vi "(SubVI)_2Dstart_BD_ver16_transfering_MultiVesselsMultiDir_OnePatch.vi"(0 "Master Ctr (Ctr0)":tag, 1 "Master Ctr Terminal (PFI0)":tag, 2 "Galvo Hardware":T2, 3 "Camera Hardware":T1, 4 "input cluster":T3, 5 "error in (no error)":errorcluster, 6 "B-Scan Frequency":dbl=100.0, 7 "A-scans per Image":u32, 8 "Camera Delay (us)":dbl format="%.6f", 9 "A-scans per Cross Section":u32, 11 "Galvo Trigg per Cross Section":u32) -> (13 "Image Size":u32, 14 "Master Ctr Task Out":refnum<k21>, 15 "Galvo AO Task Out":refnum<k21>, 16 "Camera Ctr Task Out":refnum<k21>, 17 "Galvo Ctr Task Out":refnum<k21>, 18 "output cluster for DLL":T3, 19 "AO Err Out":errorcluster)   [LabVIEW 2019]
uses:
  <vilib>/DAQmx/write.llb/DAQmx Write (Analog 2D DBL NChan NSamp).vi
  <vilib>/DAQmx/create/channels.llb/DAQmx Create Channel (CO-Pulse Generation-Frequency).vi
  <vilib>/DAQmx/configure/timing.llb/DAQmx Timing (Implicit).vi
  <vilib>/DAQmx/configure/trigger.llb/DAQmx Start Trigger (Digital Edge).vi
  <vilib>/DAQmx/create/channels.llb/DAQmx Create Channel (AO-Voltage-Basic).vi
  <vilib>/DAQmx/configure/timing.llb/DAQmx Timing (Sample Clock).vi
  <vilib>/DAQmx/miscellaneous.llb/DAQmx Fill In Error Info.vi
  <resource>/objmgr/daqmx.rc
panel:
  out "B-Scan Frequency 2":dbl
  in  "counter":tag
  out "error out":errorcluster
  out "task out":refnum<k21>
  in  "2D frequency":i16
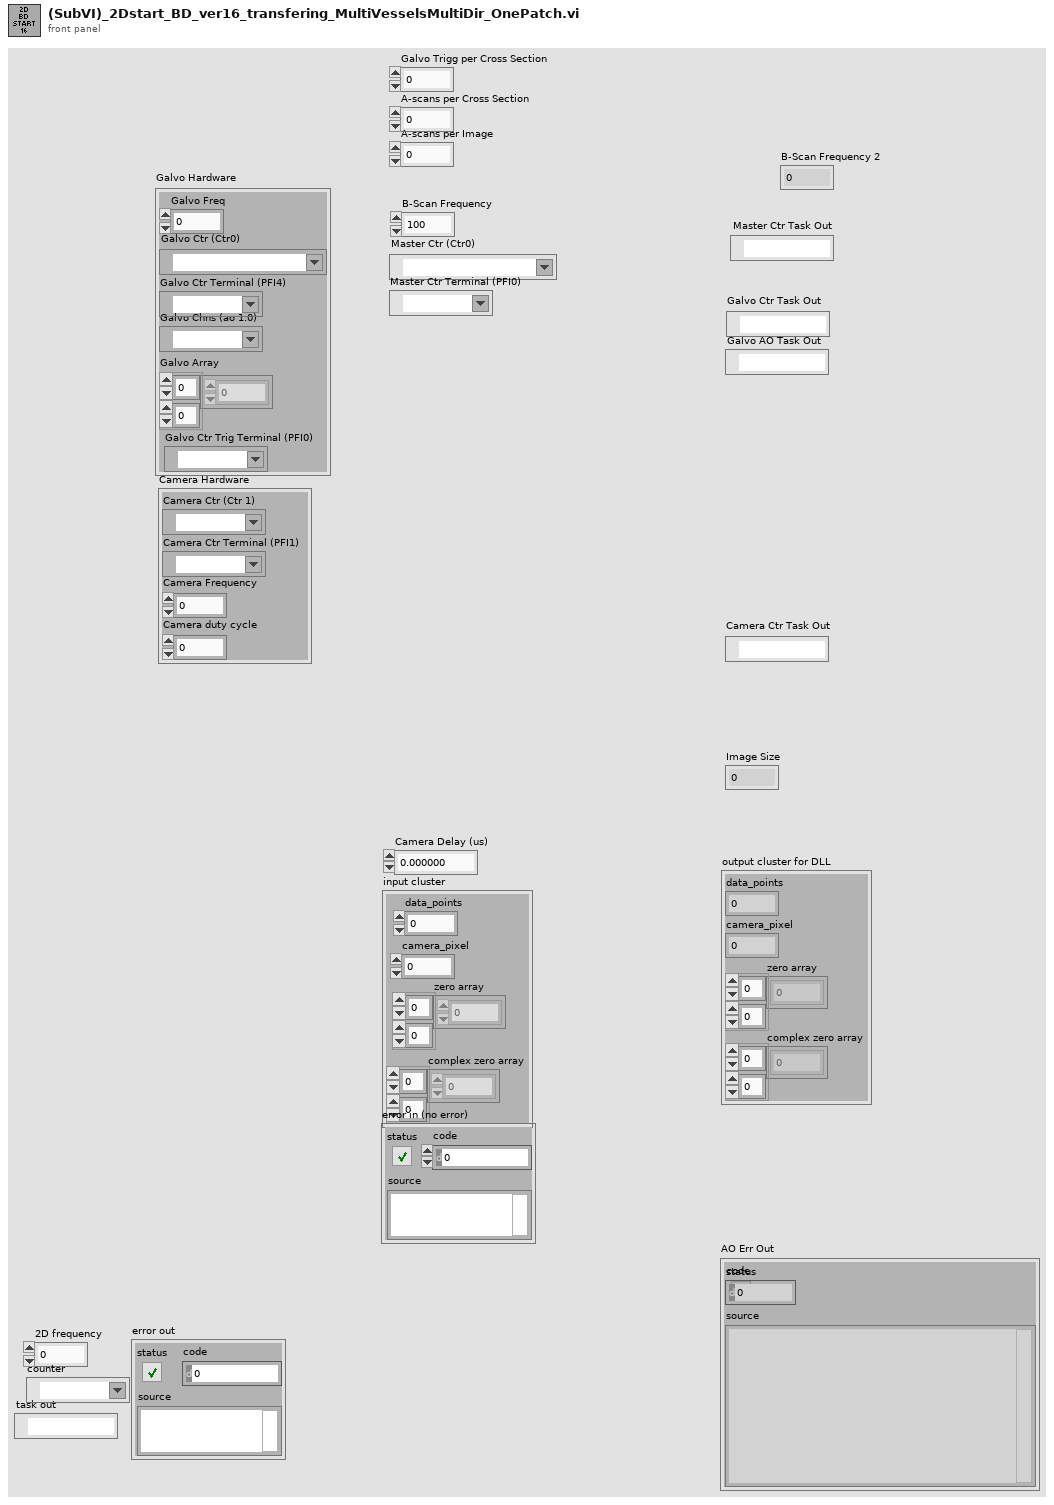
[diagram p1: front panel]
types:
  T1 = cluster{"Camera Ctr (Ctr 1)":tag, "Camera Ctr Terminal (PFI1)":tag, "Camera Frequency":dbl, "Camera duty cycle":dbl}
  T2 = cluster{"Galvo Array":dbl[][], "Galvo Chns (ao 1:0)":tag, "Galvo Ctr (Ctr0)":tag, "Galvo Ctr Terminal (PFI4)":tag, "Galvo Freq":dbl, "Galvo Ctr Trig Terminal (PFI0)":tag}
  T3 = cluster{"data_points":i32, "camera_pixel":i32, "zero array":dbl[][], "complex zero array":dbl[][]}
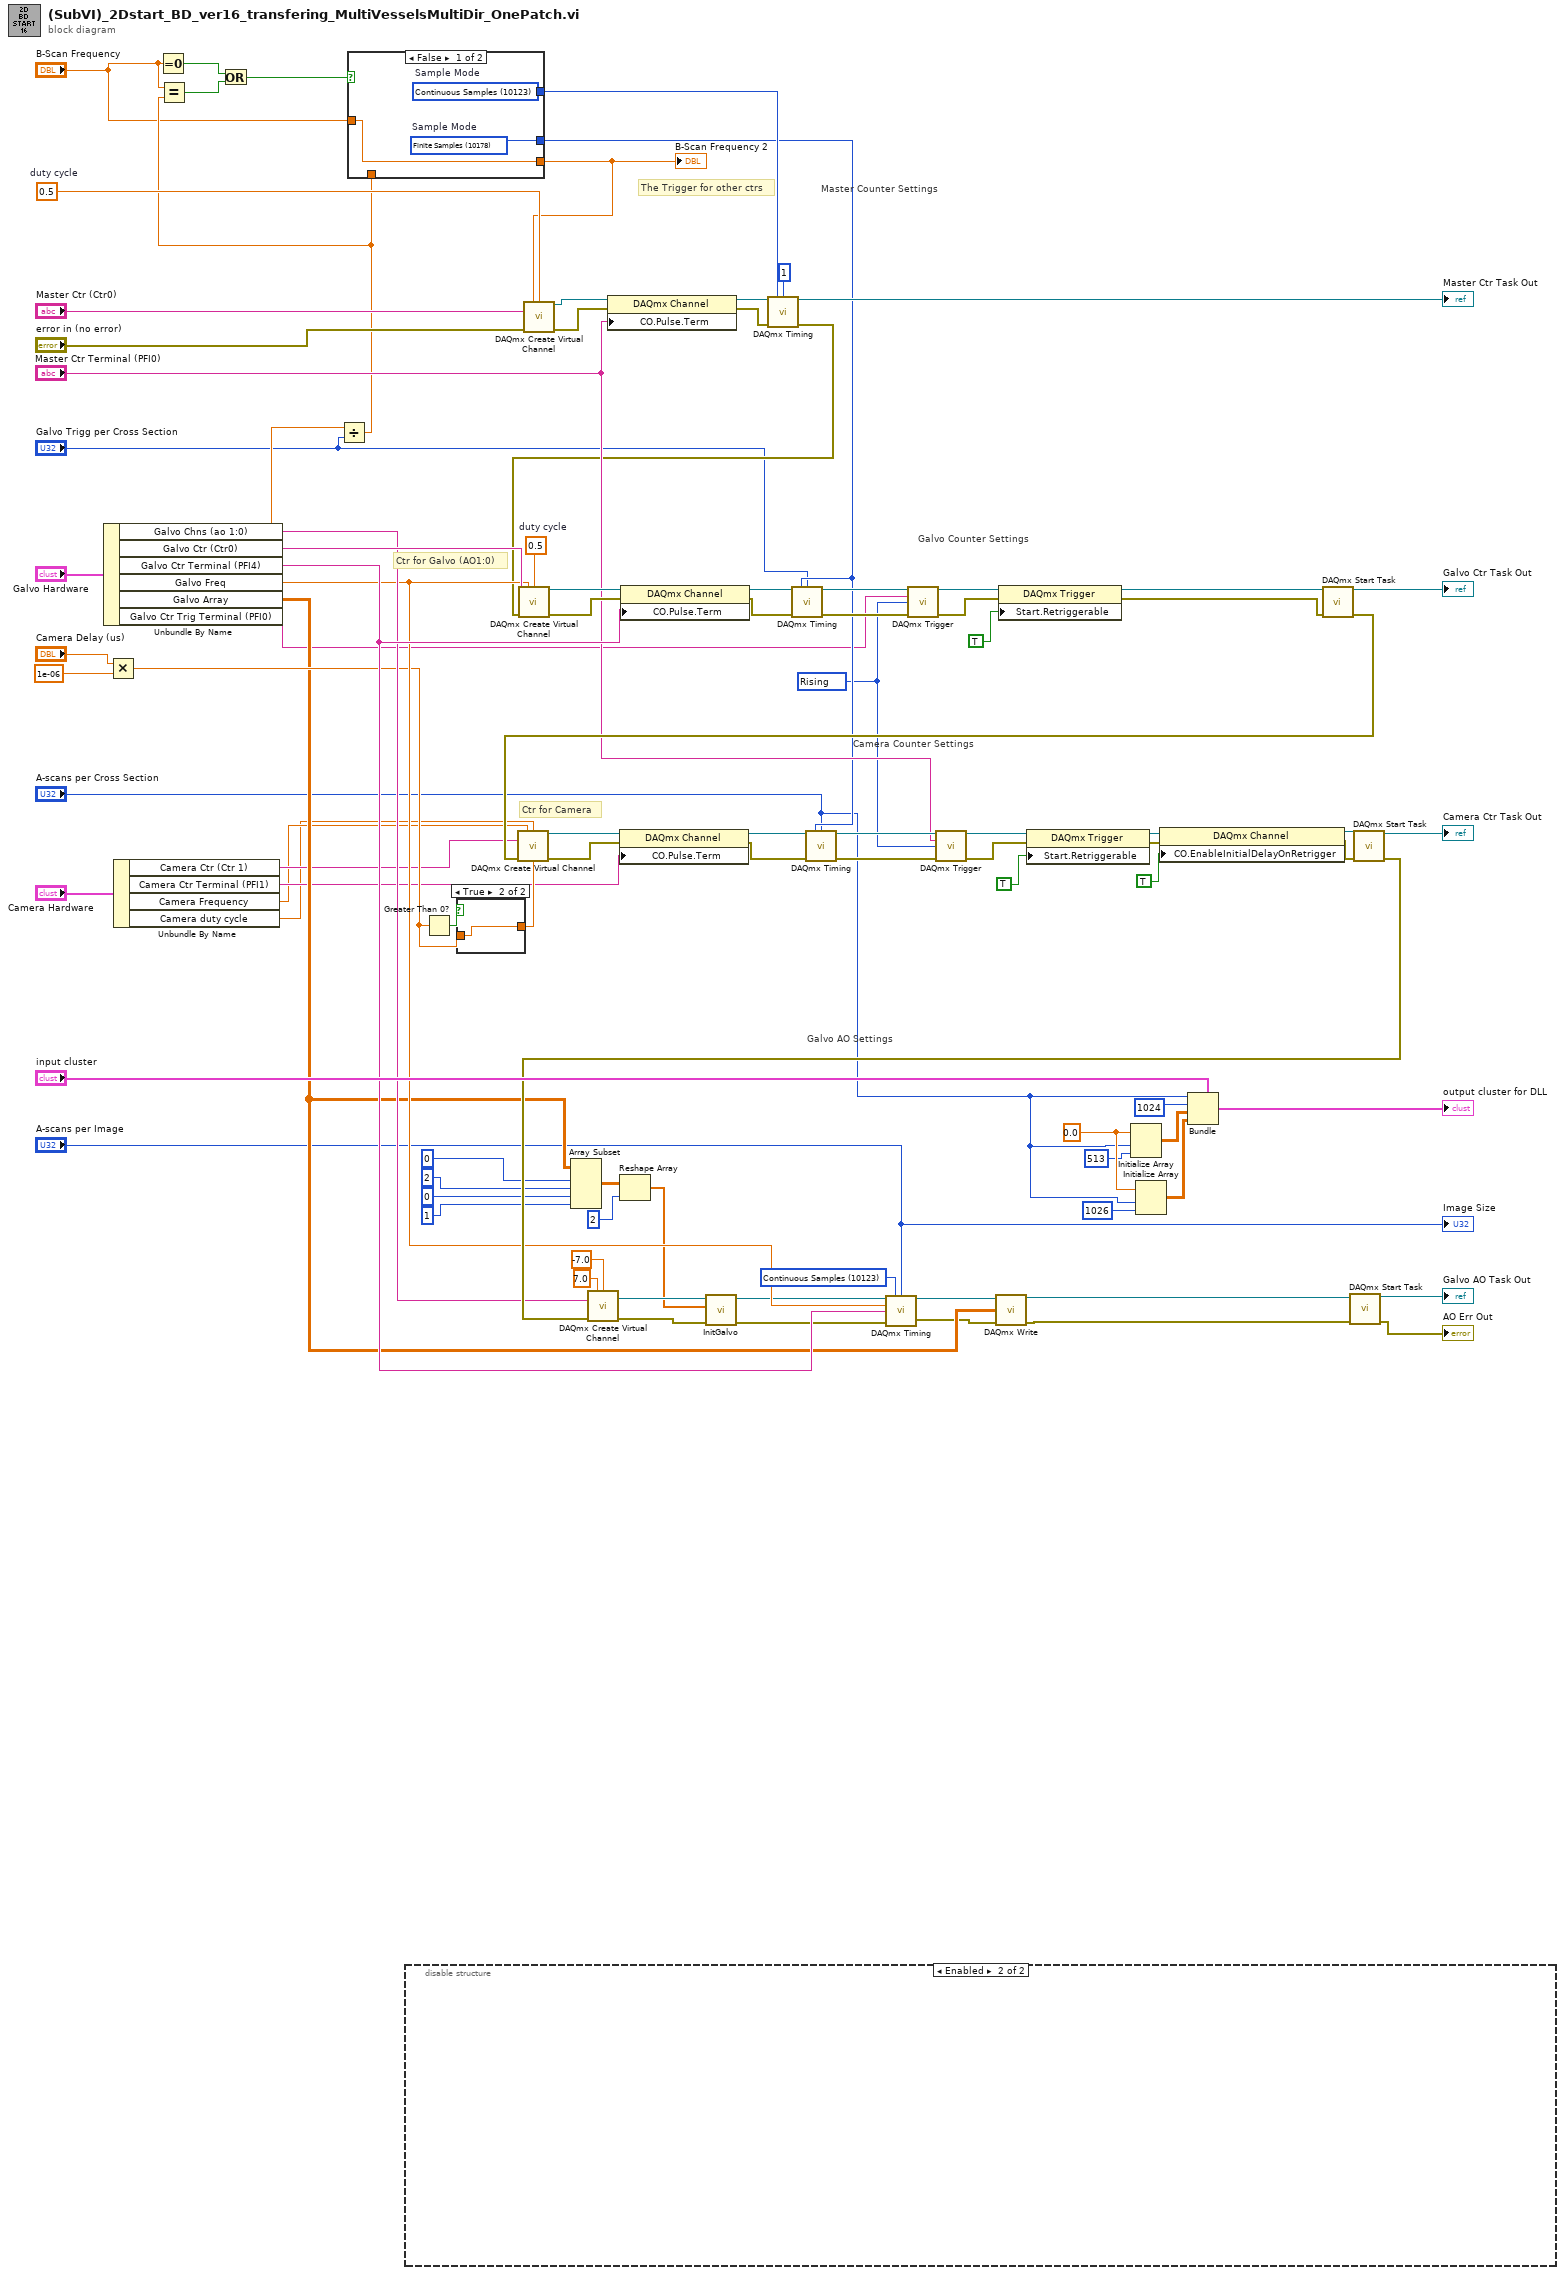
[diagram p0: block diagram]
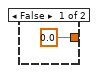
[diagram p2: hidden frame]
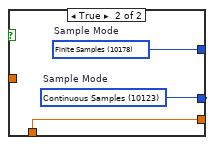
[diagram p3: hidden frame]
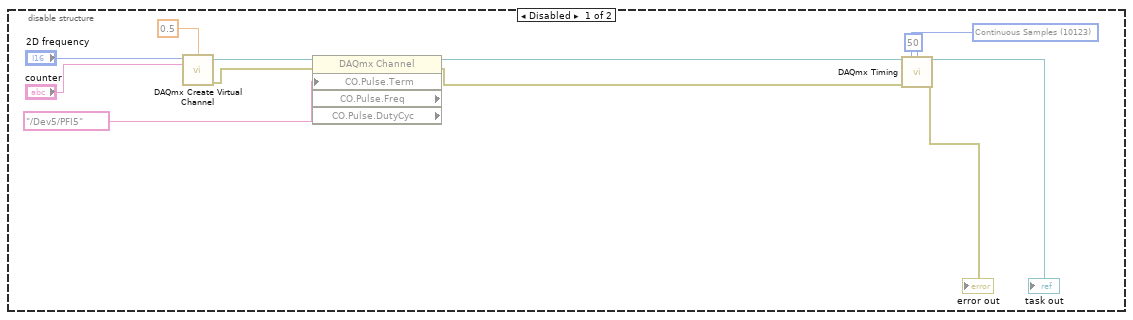
[diagram p4: hidden frame]
diagram:
  w27 = 0.0 ("element")
  w22 = 10123 items=["Finite Samples"=10178, "Continuous Samples"=10123, "Hardware Timed Single Point"=12522] ("sample mode")
  w46 = 10280 items=["Rising"=10280, "Falling"=10171] ("edge")
  w89 = 0.5  # duty cycle
  w94 = 0.5  # duty cycle
  # "Galvo AO Settings"
  # "Camera Counter Settings"
  # "Galvo Counter Settings"
  # "Master Counter Settings"
  # "Ctr for Camera"
  # "Ctr for Galvo (AO1:0)"
  # "The Trigger for other ctrs"
  n1 = Unbundle By Name("Galvo Hardware") -> ("Galvo Chns (ao 1:0)"=w66:tag, "Galvo Ctr (Ctr0)"=w68:tag, "Galvo Ctr Terminal (PFI4)"=w69:tag, "Galvo Freq"=w58:dbl, "Galvo Array"=w45:dbl[][], "Galvo Ctr Trig Terminal (PFI0)"=w7:tag)
  n2 = Multiply(x="Camera Delay (us)", y=1e-06) -> (x*y=w53:dbl)
  n3 = Unbundle By Name("Camera Hardware") -> ("Camera Ctr (Ctr 1)"=w43:tag, "Camera Ctr Terminal (PFI1)"=w42:tag, "Camera Frequency"=w41:dbl, "Camera duty cycle"=w40:dbl)
  n4 = Equal To 0?(x="B-Scan Frequency") -> (x = 0?=w37:bool)
  n5 = Divide(x=w58, y="Galvo Trigg per Cross Section") -> (x/y=w39:dbl)
  n6 = Equal?(x="B-Scan Frequency", y=w39) -> (x = y?=w36:bool)
  n7 = Or(x=w37, y=w36) -> (x .or. y?=w35:bool)
  n8 = case shown="False" w35 {
    tunnel: "B-Scan Frequency" -> [w101 _]
    tunnel: [w101 w104] -> w50
    tunnel: w39 -> [_ w104]
    tunnel: [w100 w103] -> w49
    tunnel: [w99 w102] -> w47
    frame False {
      w99 = 10178 items=["Finite Samples"=10178, "Continuous Samples"=10123, "Hardware Timed Single Point"=12522]  # Sample Mode
      w100 = 10123 items=["Finite Samples"=10178, "Continuous Samples"=10123, "Hardware Timed Single Point"=12522]  # Sample Mode
    }
    frame True {
      w102 = 10123 items=["Finite Samples"=10178, "Continuous Samples"=10123, "Hardware Timed Single Point"=12522]  # Sample Mode
      w103 = 10178 items=["Finite Samples"=10178, "Continuous Samples"=10123, "Hardware Timed Single Point"=12522]  # Sample Mode
    }
  }
  "B-Scan Frequency 2" <- w50
  n9 = disable-structure shown="Enabled" {
    frame Disabled {
      w113 = 10123 items=["Finite Samples"=10178, "Continuous Samples"=10123, "Hardware Timed Single Point"=12522] ("sample mode")
      n10 = call-poly <vilib>:"DAQmx Create Virtual Channel.vi"("frequency"="2D frequency", "duty cycle"=0.5, "counter"="counter") -> ("task out"=w109:refnum<k21>, "error out"=w108:errorcluster)  [unwired: 6 in, 5 out]
      n11 = property class="DAQmx Channel" props=["CO.Pulse.Term", "CO.Pulse.Freq", "CO.Pulse.DutyCyc"](reference=w109, error in=w108, "CO.Pulse.Term"=tag "/Dev5/PFI5") -> (reference out=w107:refnum<k21>, error out=w106:errorcluster)  [unwired: 2 out]
      n12 = call-poly <vilib>:"DAQmx Timing.vi"("task/channels in"=w107, "sample mode"=w113, "samples per channel"=50, "error in"=w106) -> ("task out"=→"task out":refnum<k21>, "error out"=→"error out":errorcluster)  [unwired: 2 in, 8 out]
    }
    frame Enabled {
    }
  }
  n13 = Greater Than 0?(x=w53) -> (x > 0?=w57:bool)
  n14 = case shown="True" w57 {
    tunnel: w53 -> [_ w118]
    tunnel: [0.0 ("Camera Delay") w118] -> w56
    frame False {
    }
    frame True {
    }
  }
  n15 = call-poly <vilib>:"DAQmx Create Virtual Channel.vi"("frequency"=w50, "duty cycle"=w94, "counter"="Master Ctr (Ctr0)", "error in"="error in (no error)") -> ("task out"=w97:refnum<k21>, "error out"=w96:errorcluster)  [unwired: 10 in]
  n16 = Array Subset(array=w45, index (row)=0 ("index"), length (row)=2 ("length"), index (col)=0 ("index"), length (col)=1 ("length")) -> (w17:dbl[][])
  n17 = property class="DAQmx Channel"(reference=w97, error in=w96, "CO.Pulse.Term"="Master Ctr Terminal (PFI0)") -> (reference out=w93:refnum<k21>, error out=w92:errorcluster)
  n18 = Reshape Array(w17, 2 ("dimension size")) -> (w12:dbl[])
  n19 = call-poly <vilib>:"DAQmx Timing.vi"("task/channels in"=w93, "sample mode"=w49, "samples per channel"=1, "error in"=w92) -> ("task out"=→"Master Ctr Task Out":refnum<k21>, "error out"=w52:errorcluster)  [unwired: 10 in]
  n20 = call-poly <vilib>:"DAQmx Create Virtual Channel.vi"("frequency"=w58, "duty cycle"=w89, "counter"=w68, "error in"=w52) -> ("task out"=w91:refnum<k21>, "error out"=w90:errorcluster)  [unwired: 10 in]
  n21 = property class="DAQmx Channel"(reference=w91, error in=w90, "CO.Pulse.Term"=w69) -> (reference out=w78:refnum<k21>, error out=w77:errorcluster)
  n22 = call-poly <vilib>:"DAQmx Timing.vi"("task/channels in"=w78, "sample mode"=w47, "samples per channel"="Galvo Trigg per Cross Section", "error in"=w77) -> ("task out"=w76:refnum<k21>, "error out"=w75:errorcluster)  [unwired: 10 in]
  n23 = call-poly <vilib>:"DAQmx Trigger.vi"("task/channels in"=w76, "source"=w7, "edge"=w46, "error in"=w75) -> ("task out"=w87:refnum<k21>, "error out"=w88:errorcluster)  [unwired: 10 in]
  n24 = property class="DAQmx Trigger"(reference=w87, error in=w88, "Start.Retriggerable"=TRUE) -> (reference out=w6:refnum<k21>, error out=w5:errorcluster)
  n25 = Initialize Array(w27, "A-scans per Cross Section", 513 ("dimension size")) -> (w25:dbl[][])
  n26 = Initialize Array(w27, "A-scans per Cross Section", 1026 ("dimension size")) -> (w26:dbl[][])
  n27 = Bundle(cluster="input cluster", "data_points"="A-scans per Cross Section", "camera_pixel"=1024, "zero array"=w25, "complex zero array"=w26) -> (→"output cluster for DLL":T3)
  n28 = call <vilib>:"DAQmx Start Task.vi"("task/channels in"=w6, "error in"=w5) -> ("task out"=→"Galvo Ctr Task Out":refnum<k21>, "error out"=w70:errorcluster)  [unwired: 12 in]
  n29 = call-poly <vilib>:"DAQmx Create Virtual Channel.vi"("frequency"=w41, "duty cycle"=w40, "counter"=w43, "error in"=w70, "initial delay"=w56) -> ("task out"=w84:refnum<k21>, "error out"=w83:errorcluster)  [unwired: 9 in]
  n30 = property class="DAQmx Channel"(reference=w84, error in=w83, "CO.Pulse.Term"=w42) -> (reference out=w74:refnum<k21>, error out=w73:errorcluster)
  n31 = call-poly <vilib>:"DAQmx Timing.vi"("task/channels in"=w74, "sample mode"=w47, "samples per channel"="A-scans per Cross Section", "error in"=w73) -> ("task out"=w72:refnum<k21>, "error out"=w71:errorcluster)  [unwired: 10 in]
  n32 = call-poly <vilib>:"DAQmx Trigger.vi"("task/channels in"=w72, "source"="Master Ctr Terminal (PFI0)", "edge"=w46, "error in"=w71) -> ("task out"=w81:refnum<k21>, "error out"=w82:errorcluster)  [unwired: 10 in]
  n33 = property class="DAQmx Trigger"(reference=w81, error in=w82, "Start.Retriggerable"=TRUE) -> (reference out=w64:refnum<k21>, error out=w63:errorcluster)
  n34 = property class="DAQmx Channel"(reference=w64, error in=w63, "CO.EnableInitialDelayOnRetrigger"=TRUE) -> (reference out=w61:refnum<k21>, error out=w60:errorcluster)
  n35 = call <vilib>:"DAQmx Start Task.vi"("task/channels in"=w61, "error in"=w60) -> ("task out"=→"Camera Ctr Task Out":refnum<k21>, "error out"=w67:errorcluster)  [unwired: 12 in]
  n36 = call-poly <vilib>:"DAQmx Create Virtual Channel.vi"("maximum value"=7.0, "minimum value"=-7.0, "physical channels"=w66, "error in"=w67) -> ("task out"=w13:refnum<k21>, "error out"=w16:errorcluster)  [unwired: 5 in, 5 out]
  n37 = call "InitGalvo.vi"("error in"=w16, "Output Array"=w12, "task/channels in"=w13) -> ("error out"=w15:errorcluster, "task out"=w14:refnum<k21>)  [unwired: 7 in]
  n38 = call-poly <vilib>:"DAQmx Timing.vi"("task/channels in"=w14, "sample mode"=w22, "samples per channel"="A-scans per Image", "rate"=w58, "source"=w69, "error in"=w15) -> ("task out"=w21:refnum<k21>, "error out"=w29:errorcluster)  [unwired: 1 in, 7 out]
  n39 = call-poly <vilib>:"DAQmx Write.vi"("task/channels in"=w21, "data"=w45, "error in"=w29) -> ("task out"=w4:refnum<k21>, "error out"=w3:errorcluster)  [unwired: 1 in, 10 out]
  n40 = call <vilib>:"DAQmx Start Task.vi"("task/channels in"=w4, "error in"=w3) -> ("task out"=→"Galvo AO Task Out":refnum<k21>, "error out"=→"AO Err Out":errorcluster)  [unwired: 12 in]
  "Image Size" <- "A-scans per Image"
